vi "MoveAwayFromBallSkill_Init.vi"(0 "object in":refnum<class "MoveAwayFromBallSkill.lvclass">, 5 "error in (no error)":errorcluster) -> (14 "object out":refnum<class "MoveAwayFromBallSkill.lvclass">, 19 "error out":errorcluster)   [LabVIEW 2020, in "MoveAwayFromBallSkill.lvclass"]
uses:
  MoveAwayFromBallSkill.lvclass
  C:/RoboIME/SSL_AI/Skill_class/Skill.lvclass
  MoveAwayFromBallSkill.lvclass/MoveAwayFromBallSkill.ctl
  Skill_class/Skill.lvclass
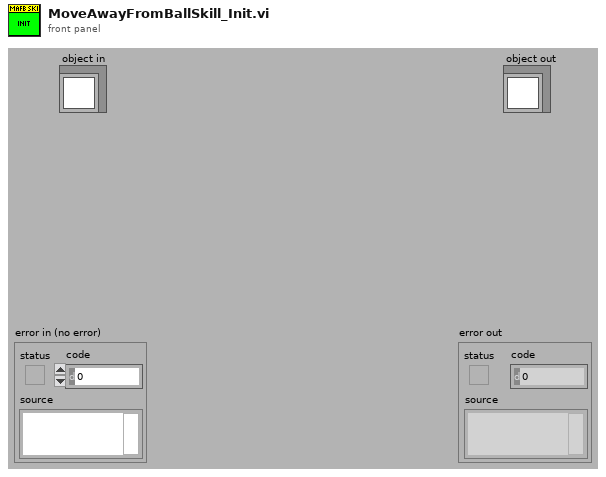
[diagram p1: front panel]
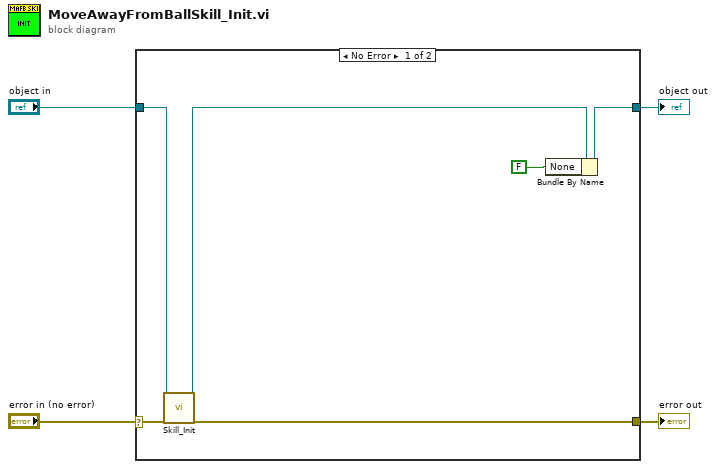
[diagram p0: block diagram]
diagram:
  n1 = case shown="No Error" "error in (no error)" {
    selector: "error in (no error)" -> [w8 w11]
    tunnel: [w10 w12] -> w4
    tunnel: "object in" -> [w6 w12]
    tunnel: [w7 w11] -> w1
    frame No Error {
      n2 = call "Skill_Init.vi"("object in"=w6, "error in (no error)"=w8) -> ("object out"=w5:refnum<class "MoveAwayFromBallSkill.lvclass">, "error out"=w7:errorcluster)  [unwired: 16 in]
      n3 = Bundle By Name(cluster=w5, "None"=FALSE) -> (w10:refnum<class "MoveAwayFromBallSkill.lvclass">)
    }
    frame Error {
    }
  }
  "object out" <- w4
  "error out" <- w1
